vi "Chapter 8 Exercise Answer.vi"() -> ()   [LabVIEW 2010]
panel:
  in  "Read Current Power":bool
  in  "Power":dbl=100.0 min=0.0 max=100.0 format="%_4f %"
  out "Device Identity":string
  out "Waveform Chart":dbl(graph)
  in  "Shutdown":bool
  out "Response":string
  in  "Set Power":bool
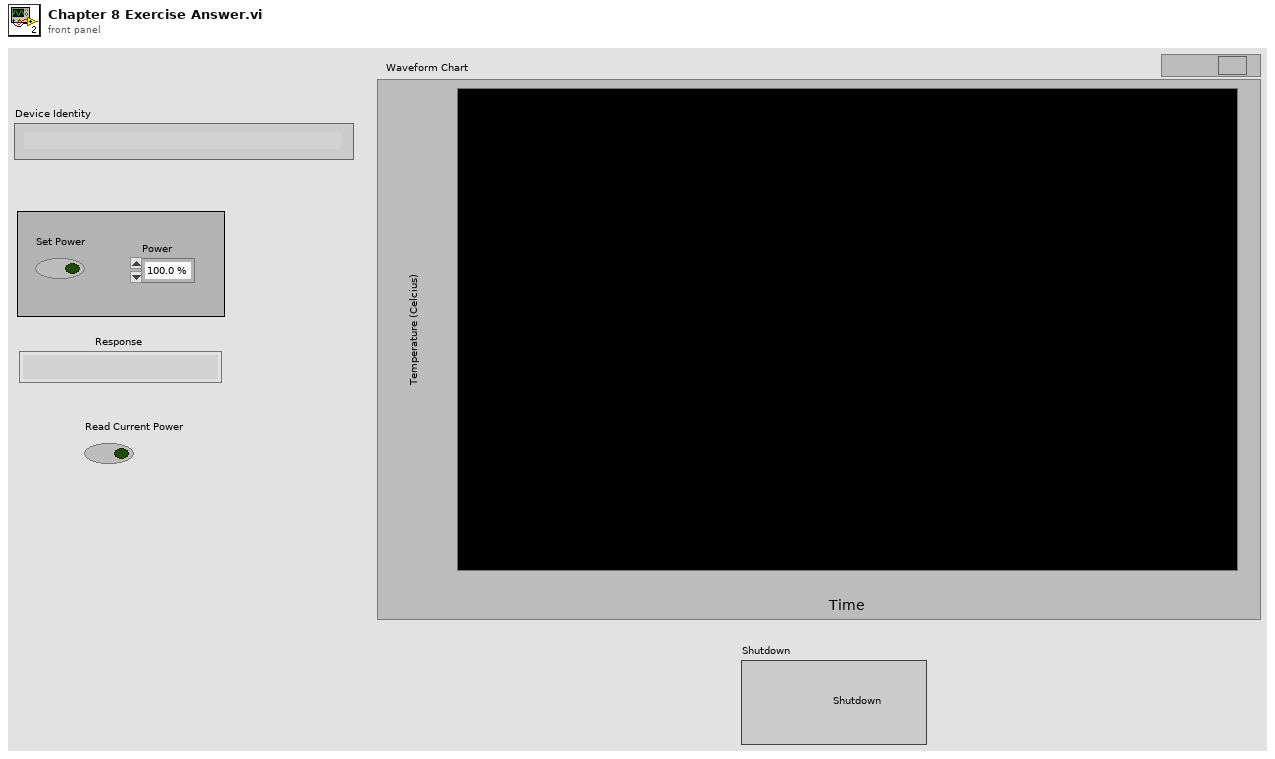
[diagram p1: front panel]
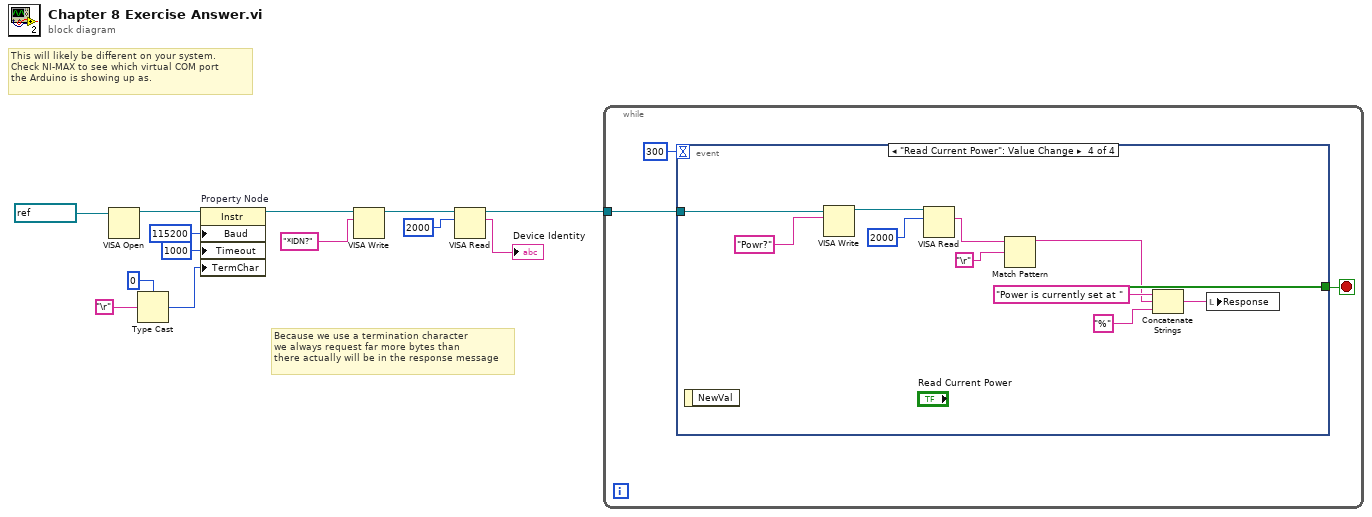
[diagram p0: block diagram]
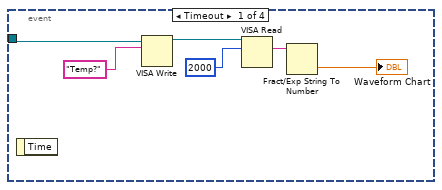
[diagram p2: hidden frame]
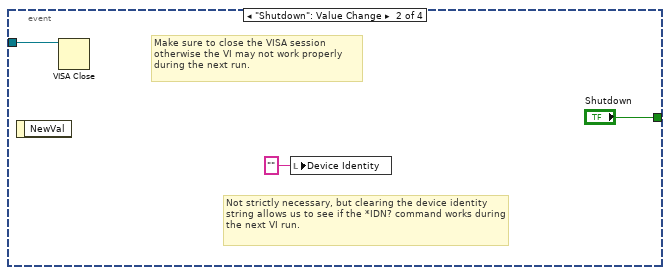
[diagram p3: hidden frame]
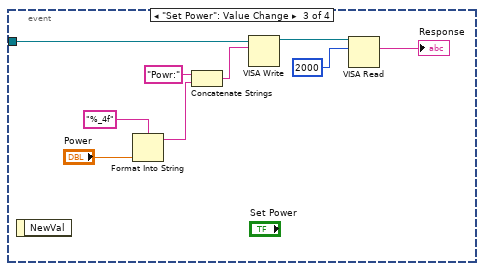
[diagram p4: hidden frame]
diagram:
  # "This will likely be different on your system.\nCheck NI-MAX to see which virtual COM port\nthe Arduino is showing up as."
  # "Because we use a termination character\nwe always request far more bytes than \nthere actually will be in the response message"
  n1 = VISA Open(VISA resource name=refnum<visa-resource-name> "COM4") -> (VISA resource name=w12:refnum<visa-resource-name>)  [unwired: 4 in, 1 out]
  n2 = Type Cast(type=u8 0 ("Message Based Settings:Termination Character"), x="\r") -> (*(type *) &x=w7:u8)
  n3 = property on="Property Node" class="Instr"(reference=w12, "Baud"=u32 115200 ("Serial Settings:Baud Rate"), "Timeout"=u32 1000 ("General Settings:Timeout Value"), "TermChar"=w7) -> (reference out=w5:refnum<visa-resource-name>)  [unwired: 1 in, 1 out]
  n4 = VISA Write(VISA resource name=w5, write buffer="*IDN?") -> (VISA resource name out=w4:refnum<visa-resource-name>)  [unwired: 1 in, 2 out]
  n5 = VISA Read(VISA resource name=w4, byte count=u32 2000) -> (VISA resource name out=w2:refnum<visa-resource-name>, read buffer=→"Device Identity":string)  [unwired: 1 in, 2 out]
  n6 = while {
    tunnel: w2 -> [w16]
    stop <- w15 stop-if-true
    n7 = event shown="[3] \"Read Current Power\": Value Change" {
      selector: _ -> [_ _ _ _]
      dyn-events: _ -> [_ _ _ _]
      timeout: 300 -> [_ _ _ _]
      tunnel: w16 -> [w20 w25 w34 w44]
      tunnel: [_ "Shutdown" _ _] -> w15
      event Timeout {
        n8 = event-data() -> ()  [unwired: 1 in, 1 out]
        n9 = VISA Write(VISA resource name=w20, write buffer="Temp?") -> (VISA resource name out=w22:refnum<visa-resource-name>)  [unwired: 1 in, 2 out]
        n10 = VISA Read(VISA resource name=w22, byte count=u32 2000) -> (read buffer=w18:string)  [unwired: 1 in, 3 out]
        n11 = Fract/Exp String To Number(string=w18) -> (number=→"Waveform Chart":dbl)  [unwired: 3 in, 1 out]
      }
      event "Shutdown": Value Change {
        # "Not strictly necessary, but clearing the device identity\nstring allows us to see if the *IDN? command works during the next VI run."
        # "Make sure to close the VISA session\notherwise the VI may not work properly\nduring the next run."
        n12 = event-data() -> ()  [unwired: 1 in, 1 out]
        n13 = VISA Close(VISA resource name=w25) -> ()  [unwired: 1 in, 1 out]
        n14 = local write "Device Identity"("") -> ()
      }
      event "Set Power": Value Change {
        n15 = event-data() -> ()  [unwired: 1 in, 1 out]
        n16 = Format Into String "Format Into String"(format string="%_4f", "Power") -> (resulting string=w29:string)  [unwired: 2 in, 1 out]
        n17 = Concatenate Strings("Powr:" ("string"), w29) -> (w27:string)
        n18 = VISA Write(VISA resource name=w34, write buffer=w27) -> (VISA resource name out=w33:refnum<visa-resource-name>)  [unwired: 1 in, 2 out]
        n19 = VISA Read(VISA resource name=w33, byte count=u32 2000) -> (read buffer=→"Response":string)  [unwired: 1 in, 3 out]
      }
      event "Read Current Power": Value Change {
        n20 = event-data() -> ()  [unwired: 1 in, 1 out]
        n21 = VISA Write(VISA resource name=w44, write buffer="Powr?" ("string")) -> (VISA resource name out=w43:refnum<visa-resource-name>)  [unwired: 1 in, 2 out]
        n22 = VISA Read(VISA resource name=w43, byte count=u32 2000) -> (read buffer=w37:string)  [unwired: 1 in, 3 out]
        n23 = Match Pattern(string=w37, regular expression="\r") -> (before substring=w35:string)  [unwired: 1 in, 3 out]
        n24 = Concatenate Strings("Power is currently set at ", w35, "%" ("string")) -> (w38:string)
        n25 = local write "Response"(w38) -> ()
      }
    }
  }
